vi "Set Database Item Body.vi"(7 "append (false)":bool, 8 "error in (no error)":errorcluster, 9 "body":string, 10 "database item id":u32, 11 "eLab in":refnum<class "PL eLabFTW Client.lvclass">) -> (0 "error out":errorcluster, 3 "eLab out":refnum<class "PL eLabFTW Client.lvclass">)   [LabVIEW 2015, in "PL eLabFTW Client.lvclass"]
doc: "Sets or appends to database item body."
uses:
  PL eLabFTW Client.lvclass
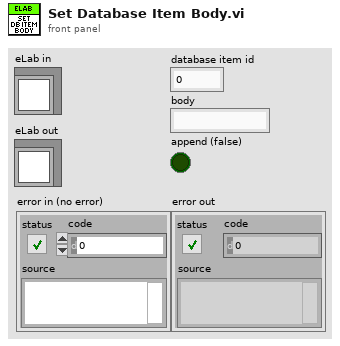
[diagram p1: front panel]
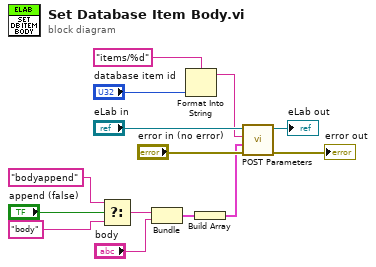
[diagram p0: block diagram]
diagram:
  n1 = Select(t="bodyappend" ("format string"), s="append (false)", f="body" ("format string")) -> (s? t:f=w4:string)
  n2 = Bundle("format string"=w4, "body"="body") -> (w2:cluster{"format string":string, "body":string})  [unwired: 1 in]
  n3 = Format Into String(format string="items/%d", "database item id") -> (resulting string=w8:string)  [unwired: 2 in, 1 out]
  n4 = Build Array(w2) -> (w1:cluster{"format string":string, "body":string}[])
  n5 = call "POST Parameters.vi"("error in (no error)"="error in (no error)", "parameters"=w1, "relative URL"=w8, "eLab in"="eLab in") -> ("error out"=→"error out":errorcluster, "eLab out"=→"eLab out":refnum<class "PL eLabFTW Client.lvclass">)  [unwired: 5 in, 1 out]
